vi "Run.vi"(8 "error in (no error)":errorcluster, 10 "OTP Cluster Out":T1, 11 "DC in":refnum<class "DC.lvclass">) -> (0 "error out":errorcluster, 1 "Parameters":cluster{"Name":string, "Value":string}[](array[cluster]), 2 "Canceled":bool, 3 "DC out":refnum<class "DC.lvclass">)   [LabVIEW 2020, in "DC.lvclass"]
doc: "This is the main test vi. It is here that the test is implemented."
uses:
  DC.lvclass
  C:/Sandbox/Git_Sandbox/WiSpry Test Framework source code (LV20)/WiSpry Test Framework/Measurements/Measurement.lvclass
  Controls/OTP_Cluster.ctl
  Controls/Run State Machine.ctl
  Measurement.lvclass/Measurement.ctl
  Devices/Controls/Change setting mode enum.ctl
  Support VI/Update parameters (array).vi
  Measurement.lvclass
  Devices/Device.lvclass
  XML Handler/XML Handler.lvclass
  Instruments/Power Supply/Power Supply.lvclass
  Instruments/Digital Multimeter/Digital Multimeter.lvclass
  Devices/PIC-device/PIC-Device.lvclass
panel:
  out "Waveform Chart":dbl[](graph)
  out "Progress":u8(slide) scale=0.0..100.0
  in  "Cancel Button":bool
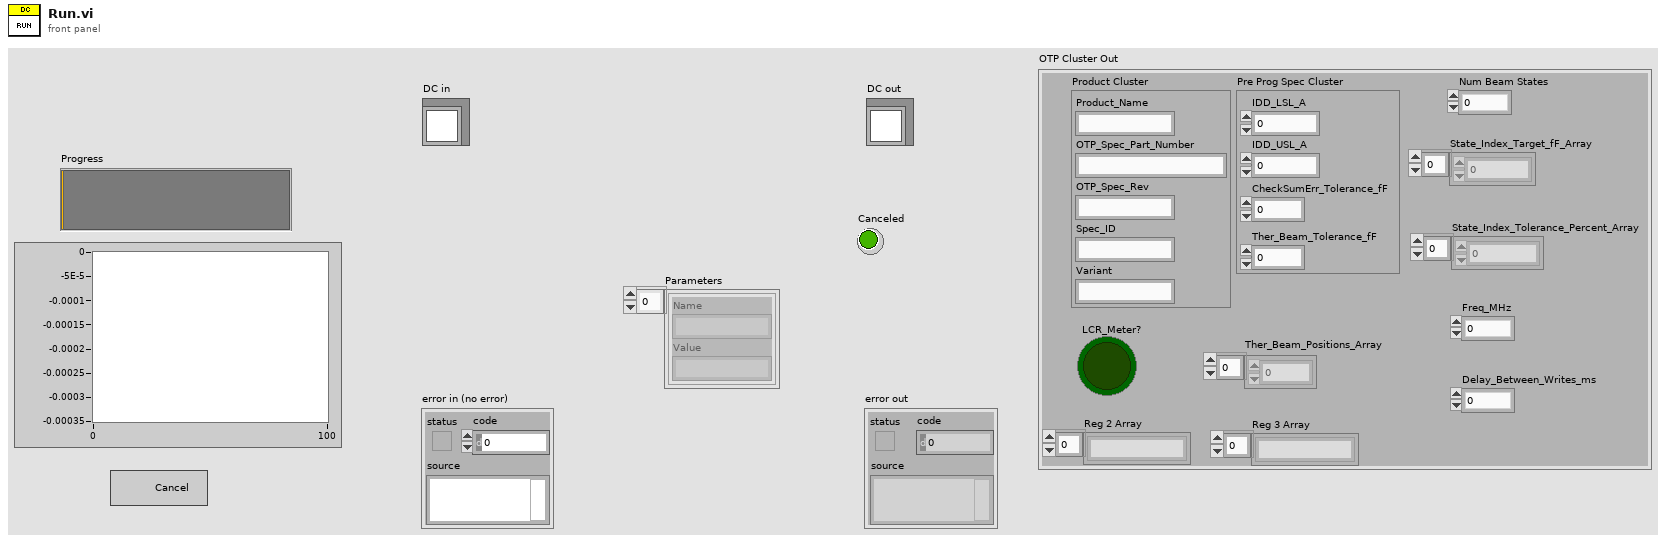
[diagram p1: front panel]
types:
  T1 = typedef "OTP_Cluster.ctl" = cluster{"Product Cluster":cluster{"Product_Name":string, "OTP_Spec_Part_Number":string, "OTP_Spec_Rev":string, "Spec_ID":string, "Variant":string}, "Pre Prog Spec Cluster":cluster{"IDD_LSL_A":dbl, "IDD_USL_A":dbl, "CheckSumErr_Tolerance_fF":dbl, "Ther_Beam_Tolerance_fF":dbl}, "LCR_Meter?":bool, "Reg 2 Array":string[], "Reg 3 Array":string[], "Num Beam States":i32, "State_Index_Target_fF_Array":dbl[], "State_Index_Tolerance_Percent_Array":dbl[], "Freq_MHz":dbl, "Delay_Between_Writes_ms":i32, "Ther_Beam_Positions_Array":i8[]}
  T2 = typedef "DC.lvclass/Run State Machine.ctl" = enum16{"Init", "Set Device", "Measure", "Done"}
  T3 = typedef "PIC-Device.lvclass/Change setting mode enum.ctl" = enum16{"Init", "Next", "Reset"}
  T4 = typedef "XML Handler.lvclass/Result Cluster.ctl" = cluster{"Name":string, "Value":string}
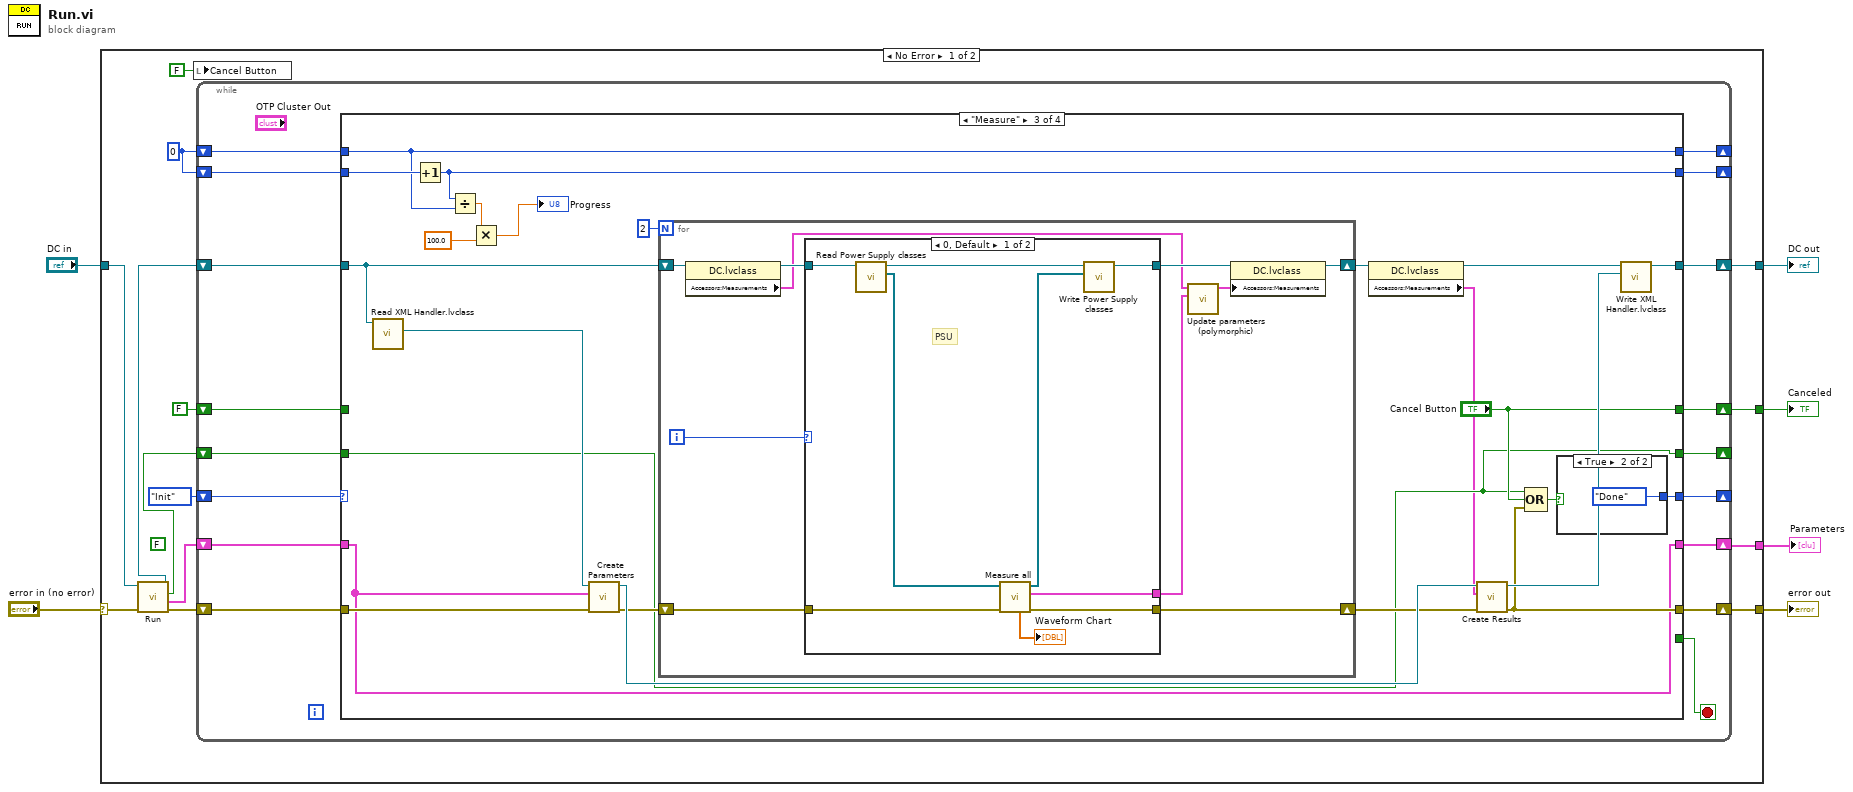
[diagram p0: block diagram]
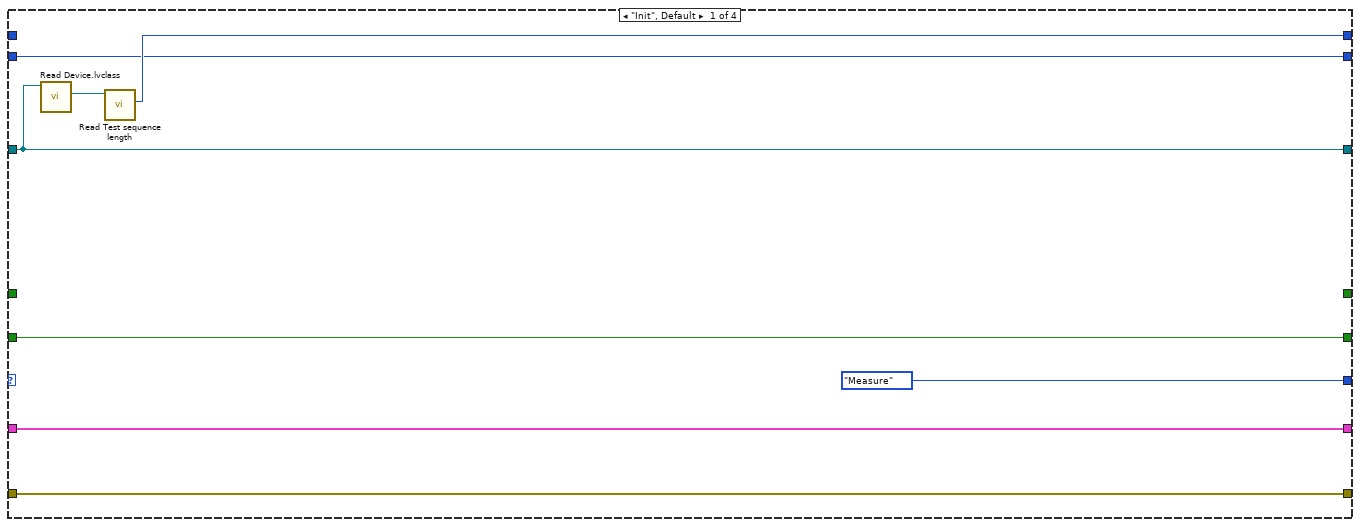
[diagram p2: hidden frame]
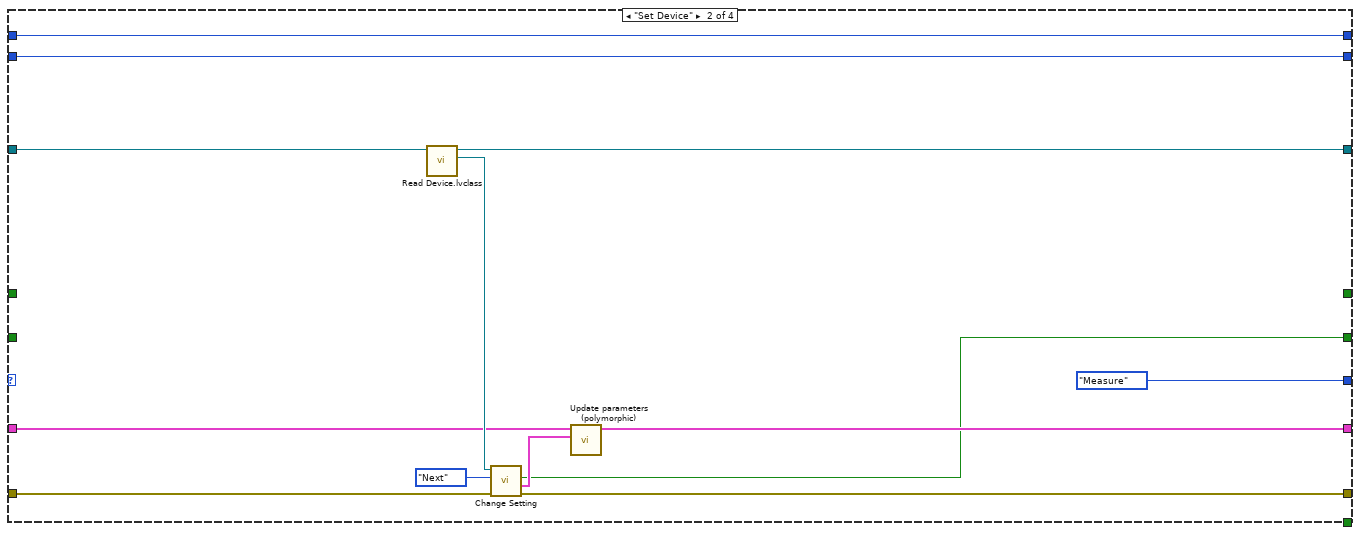
[diagram p3: hidden frame]
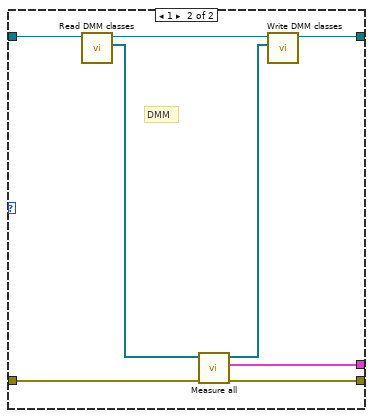
[diagram p4: hidden frame]
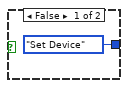
[diagram p5: hidden frame]
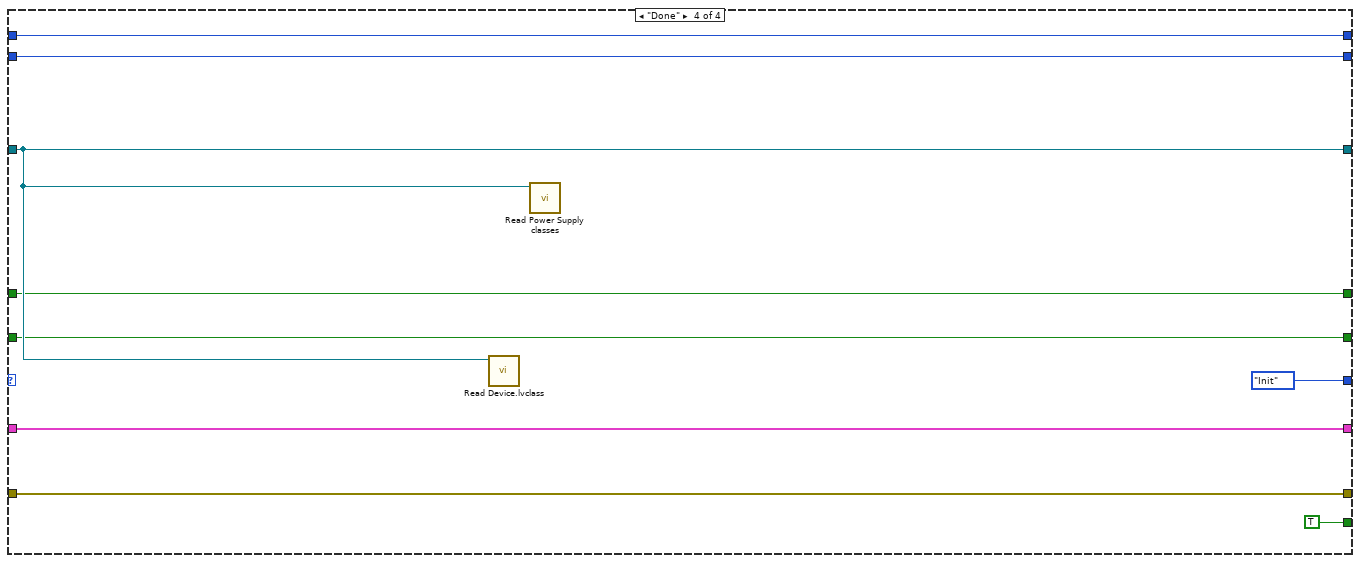
[diagram p6: hidden frame]
diagram:
  n1 = case shown="No Error" "error in (no error)" {
    selector: "error in (no error)" -> [w14 w121]
    tunnel: "DC in" -> [w10 w122]
    tunnel: [w18 _] -> w3
    tunnel: [w17 w121] -> w4
    tunnel: [w16 w122] -> w2
    tunnel: [w15 _] -> w1
    frame No Error {
      (unwired) FALSE
      w19 = 0
      n2 = call-parent "Run.vi"("error in (no error)"=w14, "Measurements in"=w10) -> ("error out"=w13:errorcluster, "Parameters"=w12:cluster{"Name":string, "Value":string}[], "Canceled"=w11:bool, "Measurements out"=w9:refnum<class "DC.lvclass">)  [unwired: 6 in]
      n3 = local write "Cancel Button"(FALSE ("Cancel Button")) -> ()
      n4 = while {
        shift-right: [w33] -> _
        shift-left: w19 -> [w35]
        shift-right: [w32] -> _
        shift-left: w19 -> [w34]
        shift-right: [w31] -> _
        shift-left: Run_State_Machine."Init" -> [w37]
        shift-right: [w29] -> w17
        shift-left: w13 -> [w30]
        shift-right: [w28] -> w16
        shift-left: w9 -> [w36]
        shift-right: [w24] -> w15
        shift-left: w12 -> [w25]
        shift-right: [w23] -> _
        shift-left: w11 -> [w22]
        shift-right: [w27] -> w18
        shift-left: FALSE ("Cancel Button") -> [w21]
        stop <- w26 stop-if-true
        n5 = case shown="\"Measure\"" w37 {
          tunnel: w36 -> [w42 w49 w63 w115]
          tunnel: w35 -> [_ w58 w81 w120]
          tunnel: w34 -> [w43 w57 w82 w118]
          tunnel: [w44 w58 w81 w120] -> w33
          tunnel: [w43 w57 w69 w118] -> w32
          tunnel: [Run_State_Machine."Measure" Run_State_Machine."Measure" w74 Run_State_Machine."Init"] -> w31
          tunnel: w30 -> [w41 w53 w65 w119]
          tunnel: [w41 w52 w70 w119] -> w29
          tunnel: [w42 w48 w76 w115] -> w28
          tunnel: [_ _ "Cancel Button" w112] -> w27
          tunnel: [_ _ _ TRUE] -> w26
          tunnel: w25 -> [w40 w51 w59 w116]
          tunnel: [w40 w50 w59 w116] -> w24
          tunnel: [w38 w46 w64 w113] -> w23
          tunnel: w22 -> [w38 _ w64 w113]
          tunnel: w21 -> [_ _ _ w112]
          frame "Init", Default {
            n6 = call "Read Device.lvclass.vi"("Measurements in"=w42) -> ("Device.lvclass"=w45:refnum<class "Device.lvclass">)  [unwired: 9 in, 1 out]
            n7 = call-dynamic "Read Test sequence length.vi"("Device in"=w45) -> ("Test sequence length"=w44:i32)  [unwired: 8 in, 2 out]
          }
          frame "Set Device" {
            n8 = call "Read Device.lvclass.vi"("Measurements in"=w49) -> ("Device.lvclass"=w55:refnum<class "Device.lvclass">, "Measurements out"=w48:refnum<class "DC.lvclass">)  [unwired: 9 in]
            n9 = call-dynamic "Change Setting.vi"("error in (no error)"=w53, "Change setting mode"=Change_setting_mode_enum."Next", "Device in"=w55) -> ("error out"=w52:errorcluster, "Changes"=w54:cluster{"Name":string, "Value":string}[], "Last setting"=w46:bool)  [unwired: 5 in, 1 out]
            n10 = call-poly "Update parameters (polymorphic).vi"("New Parameters"=w54, "Parameters"=w51) -> ("Parameters Out"=w50:cluster{"Name":string, "Value":string}[])  [unwired: 9 in]
          }
          frame "Measure" {
            n11 = call "Read XML Handler.lvclass.vi"("Measurements in"=w63) -> ("XML Handler.lvclass"=w71:refnum<class "XML Handler.lvclass">)  [unwired: 9 in, 1 out]
            n12 = Increment(x=w82) -> (x+1=w69:i32)
            n13 = Divide(x=w69, y=w81) -> (x/y=w79:dbl)
            n14 = Multiply(x=w79, y=100.0) -> (x*y=→"Progress":dbl)
            n15 = call "Create Parameters.vi"("error in (no error)"=w65, "Parameters"=w59, "XML Handler in"=w71) -> ("error out"=w68:errorcluster, "XML Handler out"=w75:refnum<class "XML Handler.lvclass">)  [unwired: 7 in]
            n16 = for {
              N: 2 -> [_]
              shift-right: [w91] -> w67
              shift-left: w68 -> [w92]
              shift-right: [w86] -> w62
              shift-left: w63 -> [w89]
              i -> [w90]
              n17 = property class="DC.lvclass"(reference=w89) -> (reference out=w88:refnum<class "DC.lvclass">, "Accessors:Measurements"=w84:cluster{"Name":string, "Value":string}[])  [unwired: 1 in, 1 out]
              n18 = case shown="0, Default" w90 {
                tunnel: [w101 w109] -> w87
                tunnel: w92 -> [w93 w106]
                tunnel: [w95 w105] -> w91
                tunnel: [w96 w102] -> w83
                tunnel: w88 -> [w100 w107]
                frame 0, Default {
                  # "PSU"
                  n19 = call-dynamic "Read Power Supply classes.vi"("Measurements in"=w100) -> ("Power Supply classes"=w98:refnum<class "Power Supply.lvclass">[], "Measurements out"=w99:refnum<class "DC.lvclass">)  [unwired: 9 in]
                  n20 = call "Measure all.vi"("error in (no error)"=w93, "Power Supplies in"=w98) -> ("error out"=w95:errorcluster, "Measurements"=w96:T4[], "Power Supplies out"=w97:refnum<class "Power Supply.lvclass">[], "Currents (A)"=→"Waveform Chart":dbl[])  [unwired: 5 in, 1 out]
                  n21 = call-dynamic "Write Power Supply classes.vi"("Power Supply classes"=w97, "Measurements in"=w99) -> ("Measurements out"=w101:refnum<class "DC.lvclass">)  [unwired: 9 in]
                }
                frame 1 {
                  # "DMM"
                  n22 = call-dynamic "Read DMM classes.vi"("Measurements in"=w107) -> ("DMM classes"=w104:refnum<class "Digital Multimeter.lvclass">[], "Measurements out"=w108:refnum<class "DC.lvclass">)  [unwired: 9 in]
                  n23 = call "Measure all.vi"("error in (no error)"=w106, "Digital Multimeters in"=w104) -> ("error out"=w105:errorcluster, "Measurements"=w102:T4[], "Digital Multimeters out"=w103:refnum<class "Digital Multimeter.lvclass">[])  [unwired: 5 in, 2 out]
                  n24 = call-dynamic "Write DMM classes.vi"("DMM classes"=w103, "Measurements in"=w108) -> ("Measurements out"=w109:refnum<class "DC.lvclass">)  [unwired: 9 in]
                }
              }
              n25 = call-poly "Update parameters (polymorphic).vi"("New Parameters"=w83, "Parameters"=w84) -> ("Parameters Out"=w85:cluster{"Name":string, "Value":string}[])  [unwired: 9 in]
              n26 = property class="DC.lvclass"(reference=w87, "Accessors:Measurements"=w85) -> (reference out=w86:refnum<class "DC.lvclass">)  [unwired: 1 in, 1 out]
            }
            n27 = property class="DC.lvclass"(reference=w62) -> (reference out=w61:refnum<class "DC.lvclass">, "Accessors:Measurements"=w60:cluster{"Name":string, "Value":string}[])  [unwired: 1 in, 1 out]
            n28 = call "Create Results.vi"("error in (no error)"=w67, "Results"=w60, "XML Handler in"=w75) -> ("error out"=w70:errorcluster, "XML Handler out"=w77:refnum<class "XML Handler.lvclass">)  [unwired: 7 in]
            n29 = Compound Arithmetic op=OR(w64, "Cancel Button", w70) -> (w73:bool)
            n30 = case shown="True" w73 {
              tunnel: [Run_State_Machine."Set Device" Run_State_Machine."Done"] -> w74
              frame False {
              }
              frame True {
              }
            }
            n31 = call "Write XML Handler.lvclass.vi"("XML Handler.lvclass"=w77, "Measurements in"=w61) -> ("Measurements out"=w76:refnum<class "DC.lvclass">)  [unwired: 9 in]
          }
          frame "Done" {
            n32 = call "Read Device.lvclass.vi"("Measurements in"=w115) -> ()  [unwired: 9 in, 2 out]
            n33 = call-dynamic "Read Power Supply classes.vi"("Measurements in"=w115) -> ()  [unwired: 9 in, 2 out]
          }
        }
      }
    }
    frame Error {
    }
  }
  "error out" <- w4
  "DC out" <- w2
  "Canceled" <- w3
  "Parameters" <- w1
